vi "LEBITplc.InitSetServices.vi"(0 "i ref in":refnum<vi>, 2 "i attribute in":T4, 5 "error in":errorcluster) -> (14 "i ref out":refnum<vi>, 16 "i attribute out":T4, 19 "error out":errorcluster)   [LabVIEW 2014, in "LEBITplc.lvlib"]
uses:
  LEBITplc.lvlib
  LEBITplc.i attribute.ctl
  CS_Core/CSSystem/CoreDefs/CoreDefs.call_type.ctl
  CS_Core/BaseProcess/BaseProcess.descriptor string definition.ctl
  CS_Core/CSSystem/CoreDefs/CoreDefs.rawDataType.ctl
  CSlibraries/UtilityLib/UtilityLib.valueStatus.ctl
  CS_Core/CSSystem/CoreLib/CoreLib.string 2 byte array.vi
  CS_Core/CSSystem/CoreLib/CoreLib.byte array 2 double.vi
  CSlibraries/UtilityLib/UtilityLib.lvlib
  CS_Core/CSSystem/CoreLib/CoreLib.lvlib
  CSlibraries-extern/DimLVEvent/LVDimInterface/LVDimInterface.lvlib
  CS_Core/BaseProcess/BaseProcess.lvlib
panel:
  in  "call cluster in":T1={"Object"="", "Selector"="", "CallType"=enum."synchronous", "Async Object"="", "Async Selector"="", "Data Descriptor"="", "Data"=[], "Error #"=0, "Expire"=0}
  in  "call cluster in":T1={"Object"="", "Selector"="", "CallType"=enum."synchronous", "Async Object"="", "Async Selector"="", "Data Descriptor"="", "Data"=[], "Error #"=0, "Expire"=0}
  in  "call cluster in":T1={"Object"="", "Selector"="", "CallType"=enum."synchronous", "Async Object"="", "Async Selector"="", "Data Descriptor"="", "Data"=[], "Error #"=0, "Expire"=0}
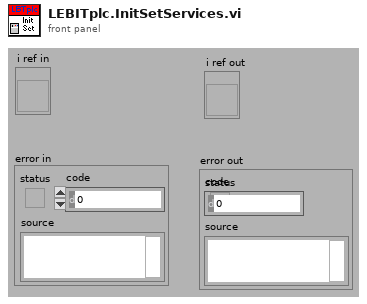
[diagram p1: front panel]
types:
  T1 = typedef "CoreDefs.call_type.ctl" = cluster{"Object":string, "Selector":string, "CallType":enum16{"simple", "synchronous", "asynchronous"}, "Async Object":string, "Async Selector":string, "Data Descriptor":T2, "Data":T3, "Error #":i32, "Expire":u32}
  T2 = typedef "BaseProcess.lvlib/BaseProcess.descriptor string definition.ctl" = string
  T3 = typedef "CoreDefs.rawDataType.ctl" = i8[]
  T4 = typedef "LEBITplc.lvlib/LEBITplc.i attribute.ctl" = cluster{"LLFLocation":string, "SetFileLocation":string, "nickNames":string[], "setValuePLCServiceID":i32[], "GUIServiceID":i32[], "monValuePLC":string[], "SetValueServiceID":i32[], "MonValueServiceID":i32[], "SetValue":dbl[][], "SetValueMin":dbl[], "SetValueMax":dbl[], "SetValueInfoServiceID":i32[], "GUINames":string[], "ListOfBases":string[], "Scale":dbl[], "Offset":dbl[], "setValuePLC":string[], "BaseName":string[], "ScaleServiceID":i32[], "OffsetServiceID":i32[], "AllPLCValues":string[], "CondSpecialArray":string[][], "CondSpecialIndex":i32[], "CondSpecialMonValue":dbl[], "RecentlyChanged":i32[], "SetFileLocationID":i32, "Dependent-Monitors":string[][], "LastLoadedFiles":string[], "IonGuideCalibLocation":string, "Monitor Dependent":string[], "Special":string[], "PLC?":bool[], "Start Date":string, "ListOfBasesServiceID":i32, "SETRA VISA resource":refnum<visa-resource-name>}
  T5 = typedef "UtilityLib.lvlib/UtilityLib.valueStatus.ctl" = enum16{"no info available", "stand by/off", "on", "warning", "alarm/malfunction", "not implemented", "user action required", "important information", "system default", "control default", "indicator default", "button default"}
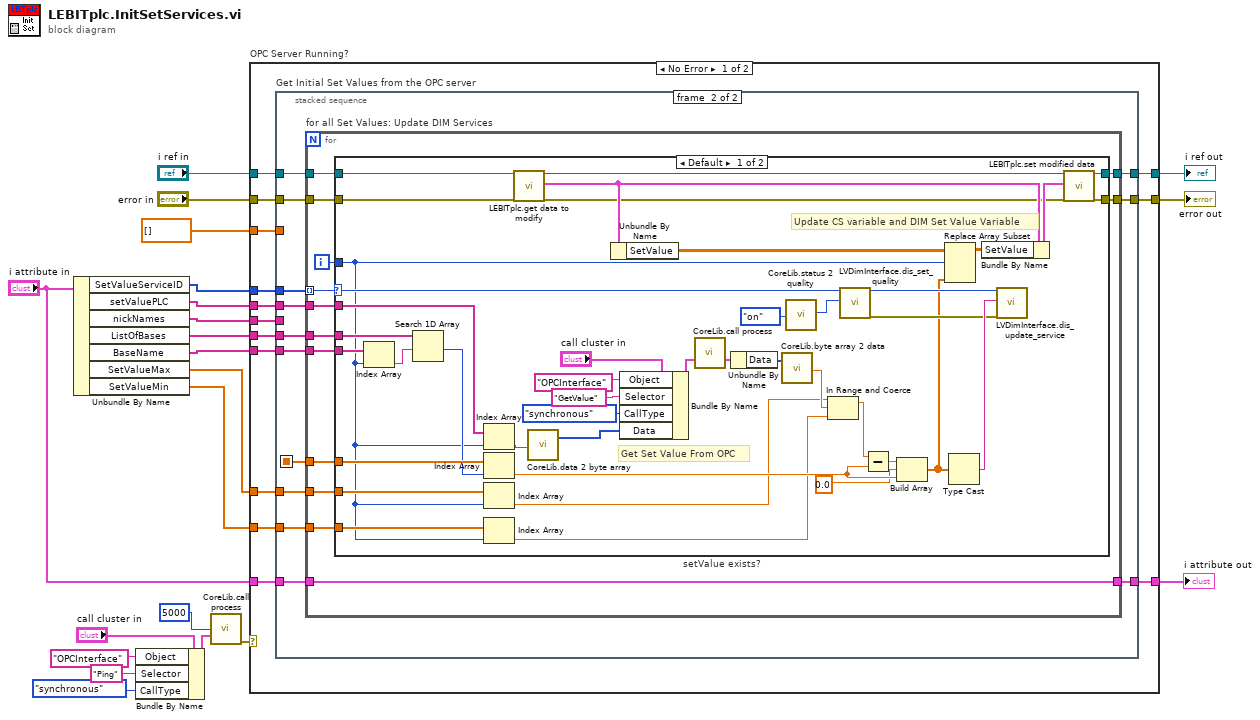
[diagram p0: block diagram]
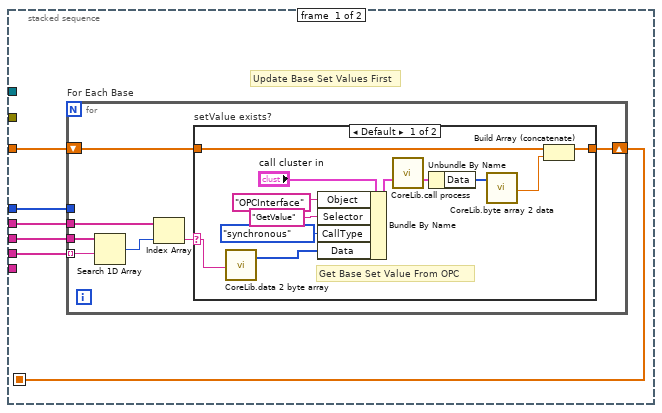
[diagram p2: hidden frame]
diagram:
  n1 = Unbundle By Name("i attribute in") -> ("SetValueServiceID"=w16:i32[], "setValuePLC"=w17:string[], "nickNames"=w12:string[], "ListOfBases"=w11:string[], "BaseName"=w10:string[], "SetValueMax"=w2:dbl[], "SetValueMin"=w1:dbl[])
  n2 = Bundle By Name(cluster="call cluster in", "Object"="OPCInterface", "Selector"="Ping" ("string"), "CallType"=enum16{"simple", "synchronous", "asynchronous"}."synchronous") -> (w6:T1)
  n3 = call "CoreLib.call process.vi"("timeout (ms)"=5000, "call cluster in"=w6) -> ("error out"=w4:errorcluster)  [unwired: 12 in, 1 out]
  n4 = case "OPC Server Running?" shown="No Error" w4 {
    selector: w4 -> [_ w132]
    tunnel: [w35 w132] -> w21
    tunnel: [w34 w134] -> w20
    tunnel: "error in" -> [w33 _]
    tunnel: "i ref in" -> [w32 w134]
    tunnel: w17 -> [w31 _]
    tunnel: w16 -> [w30 _]
    tunnel: "i attribute in" -> [w29 w133]
    tunnel: [w28 w133] -> w14
    tunnel: dbl[] [] -> [w27 _]
    tunnel: w12 -> [w26 _]
    tunnel: w11 -> [w25 _]
    tunnel: w10 -> [w24 _]
    tunnel: w2 -> [w23 _]
    tunnel: w1 -> [w22 _]
    frame No Error {
      n5 = stacked-sequence "Get Initial Set Values from the OPC server" {
        seq-local: [w36 _] -> [_ w64]
        tunnel: [_ w74] -> w35
        tunnel: [_ w73] -> w34
        tunnel: w33 -> [_ w72]
        tunnel: w32 -> [_ w71]
        tunnel: w31 -> [w38 w70]
        tunnel: w30 -> [w39 w69]
        tunnel: w29 -> [_ w68]
        tunnel: [_ w67] -> w28
        tunnel: w25 -> [w40 w66]
        tunnel: w26 -> [w41 _]
        tunnel: w27 -> [w37 _]
        tunnel: w24 -> [_ w65]
        tunnel: w23 -> [_ w63]
        tunnel: w22 -> [_ w62]
        frame #0 {
          # "Update Base Set Values First"
          n6 = for "For Each Base" {
            tunnel: w41 -> [w48]
            tunnel: w40 -> [w47] mode=indexing
            tunnel: w39 -> [_]
            tunnel: w38 -> [w46]
            shift-right: [w42] -> w36
            shift-left: w37 -> [w43]
            n7 = Search 1D Array(1D array=w48, element=w47) -> (index of element=w45:i32)  [unwired: 1 in]
            n8 = Index Array(array=w46, index=w45) -> (element=w44:string)
            n9 = case "setValue exists?" shown="Default" w44 {
              selector: w44 -> [w52 _]
              tunnel: w43 -> [w51 w61]
              tunnel: [w49 w61] -> w42
              frame Default {
                # "Get Base Set Value From OPC"
                n10 = call-poly "CoreLib.data 2 byte array.vi"("string"=w52) -> ("byteArray out"=w60:T3)  [unwired: 18 in]
                n11 = Bundle By Name(cluster="call cluster in", "Object"="OPCInterface", "Selector"="GetValue" ("string"), "CallType"=enum16{"simple", "synchronous", "asynchronous"}."synchronous", "Data"=w60) -> (w58:T1)
                n12 = call "CoreLib.call process.vi"("call cluster in"=w58) -> ("call cluster out"=w54:T1)  [unwired: 13 in, 1 out]
                n13 = Unbundle By Name(w54) -> ("Data"=w53:T3)
                n14 = call-poly "CoreLib.byte array 2 data.vi"("byteArray"=w53) -> ("d64"=w50:dbl)  [unwired: 16 in, 2 out]
                n15 = Build Array (concatenate)(w51, w50) -> (w49:dbl[])
              }
              frame "" {
              }
            }
          }
        }
        frame #1 {
          n16 = for "for all Set Values: Update DIM Services" {
            tunnel: w69 -> [w87] mode=indexing
            tunnel: w70 -> [w86]
            tunnel: w71 -> [w85]
            tunnel: w72 -> [w84]
            tunnel: [w83] -> w74
            tunnel: [w82] -> w73
            tunnel: w68 -> [w81]
            tunnel: [w81] -> w67
            tunnel: w66 -> [w78]
            tunnel: w65 -> [w79]
            tunnel: w64 -> [w77]
            tunnel: w63 -> [w76]
            tunnel: w62 -> [w75]
            i -> [w80]
            n17 = case "setValue exists?" shown="Default" w87 {
              selector: w87 -> [w117 _]
              tunnel: w86 -> [w103 _]
              tunnel: w85 -> [w115 w131]
              tunnel: w84 -> [w114 w130]
              tunnel: [w112 w130] -> w83
              tunnel: [w113 w131] -> w82
              tunnel: w80 -> [w88 _]
              tunnel: w79 -> [w102 _]
              tunnel: w78 -> [w101 _]
              tunnel: w77 -> [w99 _]
              tunnel: w76 -> [w93 _]
              tunnel: w75 -> [w92 _]
              frame Default {
                # "Update CS variable and DIM Set Value Variable"
                # "Get Set Value From OPC"
                n18 = Index Array(array=w102, index=w88) -> (element=w100:string)
                n19 = Search 1D Array(1D array=w101, element=w100) -> (index of element=w91:i32)  [unwired: 1 in]
                n20 = Index Array(array=w103, index=w88) -> (element=w104:string)
                n21 = Index Array(array=w99, index=w91) -> (element=w97:dbl)
                n22 = Index Array(array=w93, index=w88) -> (element=w94:dbl)
                n23 = Index Array(array=w92, index=w88) -> (element=w90:dbl)
                n24 = call "LEBITplc.get data to modify.vi"("i ref in"=w115, "error in (no error)"=w114) -> ("i ref out"=w106:refnum<vi>, "i attribute"=w109:T4, "error out"=w105:errorcluster)  [unwired: 14 in, 1 out]
                n25 = call-poly "CoreLib.data 2 byte array.vi"("string"=w104) -> ("byteArray out"=w123:T3)  [unwired: 18 in]
                n26 = Unbundle By Name(w109) -> ("SetValue"=w111:dbl[][])
                n27 = Bundle By Name(cluster="call cluster in", "Object"="OPCInterface", "Selector"="GetValue" ("string"), "CallType"=enum16{"simple", "synchronous", "asynchronous"}."synchronous", "Data"=w123) -> (w120:T1)
                n28 = call "CoreLib.call process.vi"("call cluster in"=w120) -> ("call cluster out"=w126:T1)  [unwired: 13 in, 1 out]
                n29 = Unbundle By Name(w126) -> ("Data"=w127:T3)
                n30 = call-poly "CoreLib.byte array 2 data.vi"("byteArray"=w127) -> ("d64"=w95:dbl)  [unwired: 16 in, 2 out]
                n31 = call "CoreLib.status 2 quality.vi"("valueStatus"=UtilityLib.valueStatus."on") -> ("quality"=w128:i32)  [unwired: 18 in]
                n32 = In Range and Coerce(upper limit=w94, x=w95, lower limit=w90) -> (coerced(x)=w89:dbl)  [unwired: 1 out]
                n33 = call "LVDimInterface.dis_set_quality.vi"("my_serviceID"=w117, "quality"=w128) -> ("my_serviceID (out)"=w118:i32, "error out"=w116:errorcluster)  [unwired: 16 in]
                n34 = Subtract(x=w89, y=w97) -> (x-y=w98:dbl)
                n35 = Build Array(w98, 0.0 ("element"), w97) -> (w110:dbl[])
                n36 = Replace Array Subset(array=w111, new element=w110, index (row)=w88) -> (w108:dbl[][])  [unwired: 1 in]
                n37 = Type Cast(x=w110) -> (*(type *) &x=w119:string)  [unwired: 1 in]
                n38 = Bundle By Name(cluster=w109, "SetValue"=w108) -> (w107:T4)
                n39 = call "LVDimInterface.dis_update_service.vi"("my_serviceID"=w118, "data"=w119, "error in (no error)"=w116) -> ()  [unwired: 14 in, 3 out]
                n40 = call "LEBITplc.set modified data.vi"("i ref in"=w106, "i attribute"=w107, "error in (no error)"=w105) -> ("i ref out"=w113:refnum<vi>, "error out"=w112:errorcluster)  [unwired: 15 in]
              }
              frame -1 {
              }
            }
          }
        }
      }
    }
    frame Error {
      # "OPC Server Not Running!"
    }
  }
  "error out" <- w21
  "i ref out" <- w20
  "i attribute out" <- w14
